vi "Oscilation.vi"() -> ()   [LabVIEW 2018]
panel:
  out "Solenóide 2":bool
  out "Solenóide 1":bool
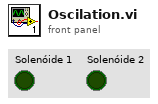
[diagram p1: front panel]
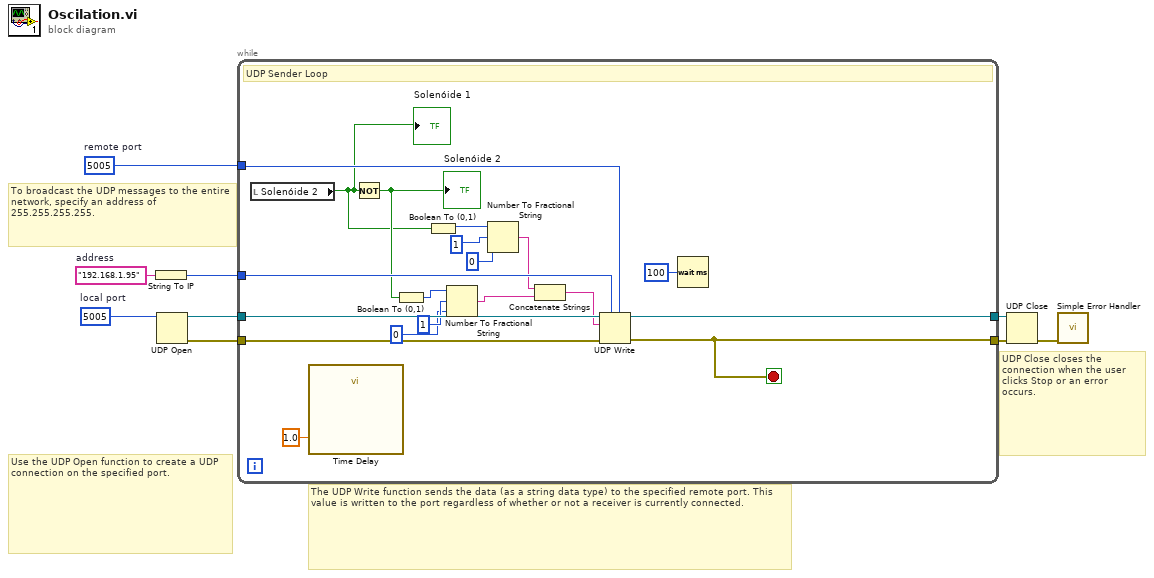
[diagram p0: block diagram]
diagram:
  w1 = u16 5005  # remote port
  w2 = u16 5005  # local port
  w7 = "192.168.1.95"  # address
  # "To broadcast the UDP messages to the entire network, specify an address of 255.255.255.255."
  # "UDP Close closes the connection when the user clicks Stop or an error occurs."
  # "The UDP Write function sends the data (as a string data type) to the specified remote port. This value is written to the port regardless of whether or not a receiver is currently connected."
  # "Use the UDP Open function to create a UDP connection on the specified port."
  n1 = String To IP(1:w7) -> (0:w5:u32)
  n2 = UDP Open(11:w2) -> (port=w4:refnum<k16>, 0:w3:errorcluster)  [unwired: 4 in, 1 out]
  n3 = while {
    tunnel: [w13] -> w8
    tunnel: w4 -> [w28]
    tunnel: w3 -> [w27]
    tunnel: [w26] -> w9
    tunnel: w5 -> [w25]
    tunnel: w1 -> [w23]
    stop <- w13 stop-if-true
    # "UDP Sender Loop"
    n4 = local read "Solenóide 2"() -> (w10:bool)
    "Solenóide 1" <- w10
    n5 = call "Time Delay"("Delay Time (s)"=1.0) -> ()  [unwired: 10 in, 1 out]
    n6 = Not(x=w10) -> (.not. x?=w11:bool)
    "Solenóide 2" <- w11
    n7 = Boolean To (0,1)(Boolean=w11) -> (0, 1=w21:i16)
    n8 = Boolean To (0,1)(Boolean=w10) -> (0, 1=w22:i16)
    n9 = Number To Fractional String(number=w21, width (-)=1, precision (6)=0) -> (F-format string=w20:string)  [unwired: 1 in]
    n10 = Number To Fractional String(number=w22, width (-)=1, precision (6)=0) -> (F-format string=w19:string)  [unwired: 1 in]
    n11 = Concatenate Strings(w19, w20) -> (w18:string)
    n12 = UDP Write(address=w25, port or service name=w23, connection ID=w28, data in=w18, 8:w27) -> (error out=w13:errorcluster, 3:w26:refnum<k16>)  [unwired: 1 in]
    n13 = Wait (ms)(milliseconds to wait=u32 100) -> ()  [unwired: 1 out]
  }
  n14 = UDP Close(connection ID=w9, 8:w8) -> (error out=w6:errorcluster)  [unwired: 1 out]
  n15 = call <vilib>:"Simple Error Handler.vi"("error in (no error)"=w6) -> ()  [unwired: 4 in, 5 out]
